vi "NICAN_CAN_Receive.vi"() -> ()   [LabVIEW 2018]
doc: "Demonstrates how to receive CAN frames via the Network Interface. \n\nTo receive frames via the Network Interface:\n- select the CAN Network Interface (i.e. CAN0, CAN1, etc.)\n- select the Baud Rate\n- select the TimeStamp mode\n- run the VI"
uses:
  <vilib>/nican/nican.llb/ncNetAttr.ctl
panel:
  out "Output Array 2":string[][](table)
  in  "interface":string(combo)="CAN0"
  in  "Baudrate":u32=125000
  in  "stop":bool
  # "See VI Info <Ctrl+I> for more information on how to use this example"
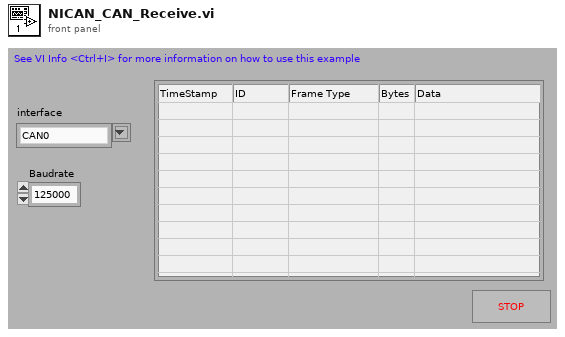
[diagram p1: front panel]
types:
  T1 = typedef "ncNetAttr.ctl" = cluster{"Start On Open":enum32{"FALSE", "TRUE"}, "Baud Rate":u32, "Read Queue Length":u32, "Write Queue Length":u32, "Standard Comparator":u32, "Standard Mask":u32, "Extended Comparator":u32, "Extended Mask":u32}
  T2 = typedef "xobjhandle.ctl" = u32
  T3 = typedef "CanFrameTimed.ctl" = cluster{"Timestamp":dbl, "ArbitrationId":u32, "IsRemote":u8, "DataLength":u8, "Data":u8[]}
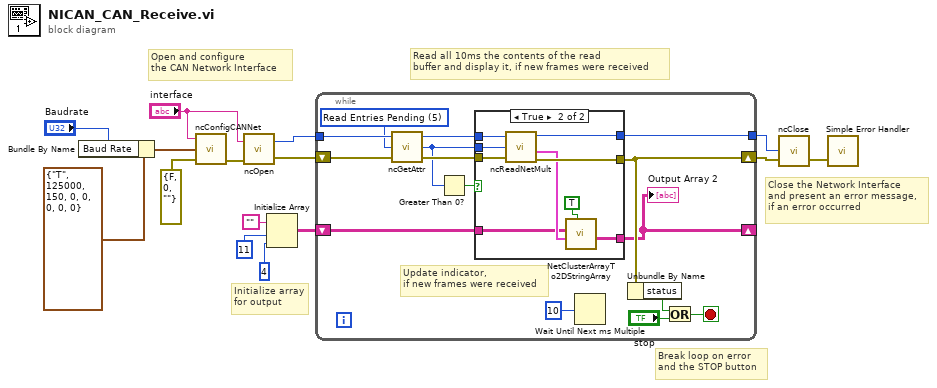
[diagram p0: block diagram]
diagram:
  # "Break loop on error \nand the STOP button"
  # "Initialize array \nfor output"
  # "Close the Network Interface \nand present an error message, \nif an error occurred"
  # "Read all 10ms the contents of the read \nbuffer and display it, if new frames were received"
  # "Open and configure \nthe CAN Network Interface"
  n1 = Bundle By Name(cluster=T1 {"Start On Open"=enum."TRUE", "Baud Rate"=125000, "Read Queue Length"=150, "Write Queue Length"=0, "Standard Comparator"=0, "Standard Mask"=0, "Extended Comparator"=0, "Extended Mask"=0} ("CAN Network Interface Config"), "Baud Rate"="Baudrate") -> (w2:T1)
  n2 = call <vilib>:"ncConfigCANNet.vi"("Error in"=errorcluster {"status"=FALSE, "code"=0, "source"=""}, "CAN Network Interface Config"=w2, "ObjName"="interface") -> ("Error out"=w12:errorcluster)  [unwired: 2 in]
  n3 = call <vilib>:"ncOpen.vi"("Error in"=w12, "ObjName"="interface") -> ("Error out"=w9:errorcluster, "ObjHandle out"=w8:T2)
  n4 = Initialize Array("", 11 ("Dimension Size"), 4 ("Dimension Size")) -> (w6:string[][])
  n5 = while {
    shift-left: w6 -> [w24]
    shift-right: [w16] -> _
    tunnel: [w25] -> w13
    tunnel: w8 -> [w23]
    shift-left: w9 -> [w22]
    shift-right: [w27] -> w15
    stop <- w26 stop-if-true
    w19 = u32 5 items=["(reserved)", "Protocol Version", "Software Version", "Object State", "(reserved)", "Read Entries Pending", "Write Entries Pending", "ReadMult Size for Notification", "Listen Only?", "Self Reception?", "Transmit Error Counter", "Receive Error Counter", "Single Shot Transmit?", "Series 2 Filter Mode", "Series 2 Mask", "Series 2 Comparator", "Serial Number", "Form Factor", "Series", "Transceiver Type", "Interface Number", "Series 2 Error/Arb Capture", "Transceiver Mode", "Transceiver External Outputs", "Transceiver External Inputs", "Start Trigger Behavior", "Log Comm Warnings", "User RTSI Frame", "Transmit Mode", "Log Start Trigger?", "Timestamp Format", "Master Timebase Rate", "Virtual Bus Timing"] ("AttrId")
    # "Update indicator, \nif new frames were received"
    n6 = call <vilib>:"ncGetAttr.vi"("Error in"=w22, "AttrId"=w19, "ObjHandle in"=w23) -> ("Error out"=w21:errorcluster, "AttrValue"=w17:u32, "ObjHandle out"=w20:T2)
    n7 = Greater Than 0?(x=w17) -> (x > 0?=w18:bool)
    n8 = case shown="True" w18 {
      tunnel: [w32 w42] -> w27
      tunnel: [w33 w40] -> w25
      tunnel: w24 -> [w31 w39]
      tunnel: w17 -> [_ w38]
      tunnel: w21 -> [w32 w37]
      tunnel: w20 -> [w33 w36]
      tunnel: [w31 w34] -> w16
      frame False {
      }
      frame True {
        n9 = call <vilib>:"ncReadNetMult.vi"("ObjHandle in"=w36, "Requested Number of Frames"=w38, "Error in"=w37) -> ("ObjHandle out"=w40:T2, "Data"=w41:T3[], "Error out"=w42:errorcluster)  [unwired: 1 out]
        n10 = call <vilib>:"NetClusterArrayTo2DStringArray.vi"("Hexadecimal?"=TRUE, "Data from ncReadNetMult"=w41, "Input Array"=w39) -> ("Output Array"=w34:string[][])  [unwired: 8 in]
      }
    }
    "Output Array 2" <- w16
    n11 = Wait Until Next ms Multiple(millisecond multiple=u32 10) -> ()  [unwired: 1 out]
    n12 = Unbundle By Name(w27) -> ("status"=w29:bool)
    n13 = Or(x=w29, y="stop") -> (x .or. y?=w26:bool)
  }
  n14 = call <vilib>:"ncClose.vi"("Error in"=w15, "ObjHandle in"=w13) -> ("Error out"=w14:errorcluster)  [unwired: 1 in]
  n15 = call <vilib>:"Simple Error Handler.vi"("error in (no error)"=w14) -> ()  [unwired: 4 in, 5 out]
